vi "Get Number.vi"(8 "error in (no error)":errorcluster, 9 "Timeout (-1)":dbl[unit], 11 "Object Ref.":refnum<class "CS++Reference.lvclass">) -> (0 "error out":errorcluster, 1 "timed out?":bool, 2 "Number":dbl, 3 "Object Ref. out":refnum<class "CS++Reference.lvclass">)   [LabVIEW 2013, in "CS++Core-Examples.lvlib" / "Example.lvclass"]
doc: "Increment Number attribute."
uses:
  Example.lvclass
  Core/Classes/CS++BaseClasses/Reference/CS++Reference.lvclass
  Example.lvclass/Example.ctl
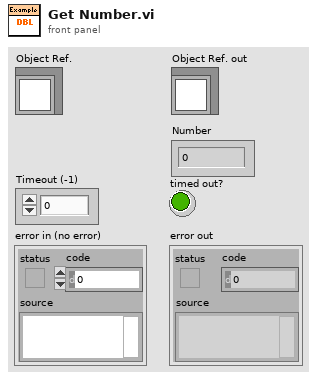
[diagram p1: front panel]
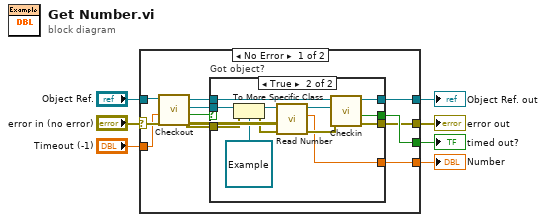
[diagram p0: block diagram]
diagram:
  n1 = case shown="No Error" "error in (no error)" {
    selector: "error in (no error)" -> [w10 w34]
    tunnel: [w11 w34] -> w6
    tunnel: [w13 w33] -> w4
    tunnel: "Object Ref." -> [w14 w33]
    tunnel: [w12 _] -> w3
    tunnel: "Timeout (-1)" -> [w9 _]
    tunnel: [w8 _] -> w1
    frame No Error {
      n2 = call "Checkout.vi"("error in (no error)"=w10, "Timeout (-1)"=w9, "Object Reference"=w14) -> ("error out"=w17:errorcluster, "Object valid??"=w16:bool, "Object"=w18:refnum<class "CS++Base.lvclass">, "Object Reference out"=w15:refnum<class "CS++Reference.lvclass">)  [unwired: 5 in]
      n3 = case "Got object?" shown="True" w16 {
        tunnel: w18 -> [_ w32]
        tunnel: w17 -> [w19 w29]
        tunnel: w15 -> [w20 w27]
        tunnel: [w20 w26] -> w13
        tunnel: [w19 w25] -> w11
        tunnel: [_ w24] -> w12
        tunnel: [_ w21] -> w8
        frame False {
        }
        frame True {
          n4 = To More Specific Class(target class=refnum<class "Example.lvclass"> refnum ("CS++Core-Examples.lvlib:Example.lvclass"), reference=w32, error in=w29) -> (specific class reference=w31:refnum<class "Example.lvclass">, error out=w28:errorcluster)
          n5 = call "Read Number.vi"("error in (no error)"=w28, "Example in"=w31) -> ("error out"=w22:errorcluster, "Number"=w21:dbl, "Example out"=w23:refnum<class "Example.lvclass">)  [unwired: 7 in]
          n6 = call "Checkin.vi"("error in (no error)"=w22, "Object"=w23, "Object Reference"=w27) -> ("error out"=w25:errorcluster, "timed out?"=w24:bool, "Object Reference out"=w26:refnum<class "CS++Reference.lvclass">)  [unwired: 6 in]
        }
      }
    }
    frame Error {
    }
  }
  "error out" <- w6
  "Object Ref. out" <- w4
  "timed out?" <- w3
  "Number" <- w1
